vi "fancy torque read T .vi"() -> (0 "timestamp":dbl, 1 "angle":dbl, 2 "field":dbl, 3 "temperature":dbl)   [LabVIEW 2017]
uses:
  read from hannes.vi
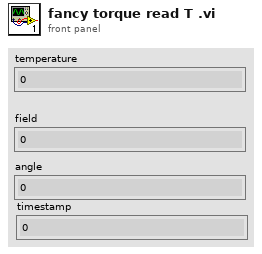
[diagram p1: front panel]
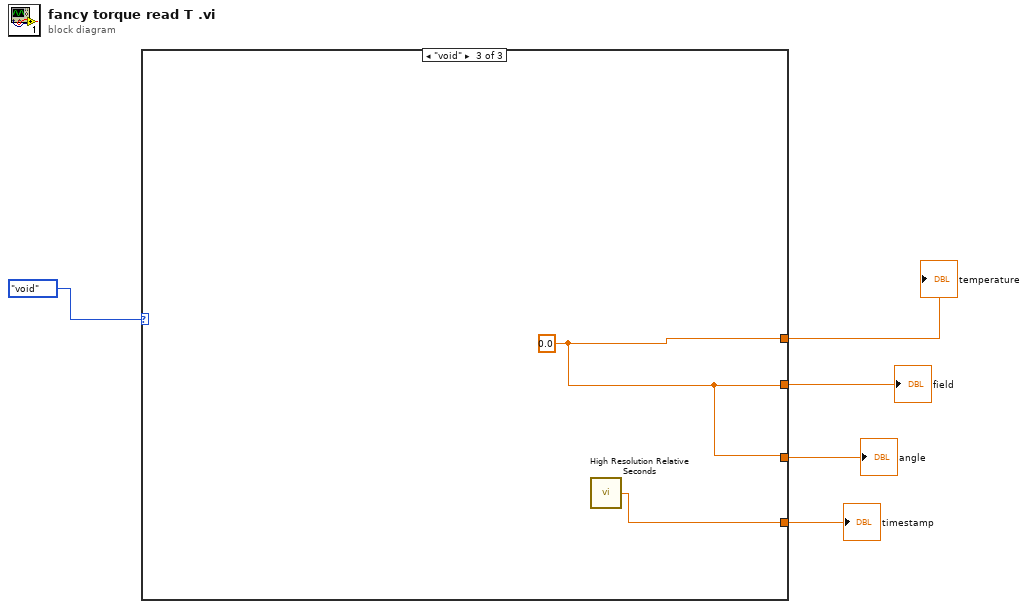
[diagram p0: block diagram]
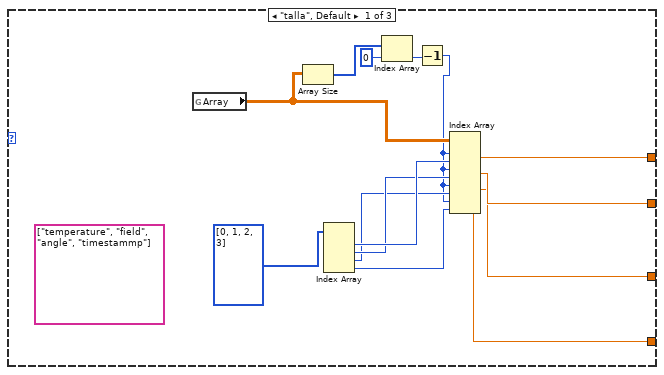
[diagram p2: hidden frame]
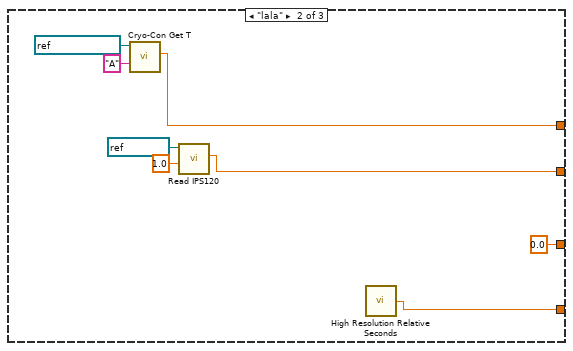
[diagram p3: hidden frame]
diagram:
  n1 = case shown="\"void\"" enum16{"talla", "lala", "void"}."void" ("kind") {
    tunnel: [w19 w25 w29] -> w5
    tunnel: [w8 w22 w29] -> w4
    tunnel: [w7 0.0 ("Numeric") w29] -> w3
    tunnel: [w6 w20 w28] -> w2
    frame "talla", Default {
      (unwired) string[] ["temperature", "field", "angle", "timestammp"]
      n2 = global read "read from hannes.vi" "Array"() -> (w13:dbl[][])
      n3 = Array Size(array=w13) -> (size(s)=w12:i32[])
      n4 = Index Array(array=i32[] [0, 1, 2, 3]) -> (element #1=w17:i32, element #2=w16:i32, element #3=w15:i32, element #4=w14:i32)  [unwired: 4 in]
      n5 = Index Array(array=w12, index=0) -> (element=w10:i32)
      n6 = Decrement(x=w10) -> (x-1=w9:i32)
      n7 = Index Array(array=w13, index (row) #1=w9, index (col) #1=w17, index (row) #2=w9, index (col) #2=w16, index (row) #3=w9, index (col) #3=w15, index (row) #4=w9, index (col) #4=w14) -> (element #1=w19:dbl, element #2=w8:dbl, element #3=w7:dbl, element #4=w6:dbl)
    }
    frame "lala" {
      n8 = call "Cryo-Con Get T.vi"("Channel"="A", "VISA Resource Name"=refnum<visa-resource-name> "CryoCon_5") -> ("Temperature"=w25:dbl)  [unwired: 6 in, 3 out]
      n9 = call "Read IPS120.vi"("Divide by"=1.0, "VISA resource name"=refnum<visa-resource-name> "COM1") -> ("Value"=w22:dbl)  [unwired: 5 in, 4 out]
      n10 = call <vilib>:"High Resolution Relative Seconds.vi"() -> ("relative seconds"=w20:dbl)
    }
    frame "void" {
      w29 = 0.0 ("Temperature")
      n11 = call <vilib>:"High Resolution Relative Seconds.vi"() -> ("relative seconds"=w28:dbl)
    }
  }
  "temperature" <- w5
  "field" <- w4
  "angle" <- w3
  "timestamp" <- w2
